vi "Excel Write Full Data Set.vi"(8 "Error In":errorcluster, 9 "CMD Step":dbl format="%#_13g", 10 "Data In":string[][](array[string]), 11 "Cells Ref In":refnum<k7>) -> (0 "Error Out":errorcluster, 3 "Cells Ref Out":refnum<k7>)   [LabVIEW 2013]
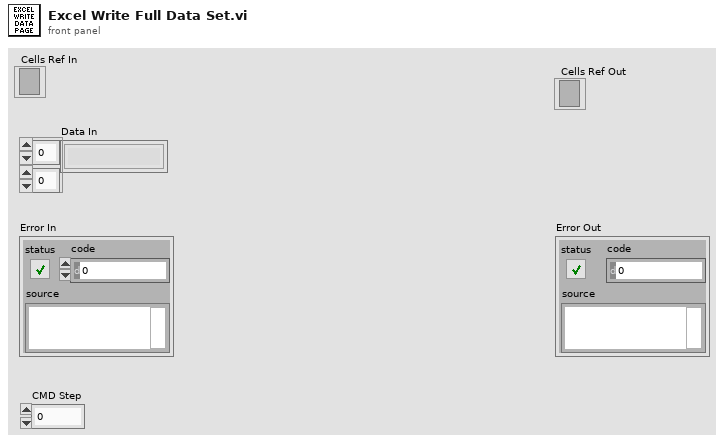
[diagram p1: front panel]
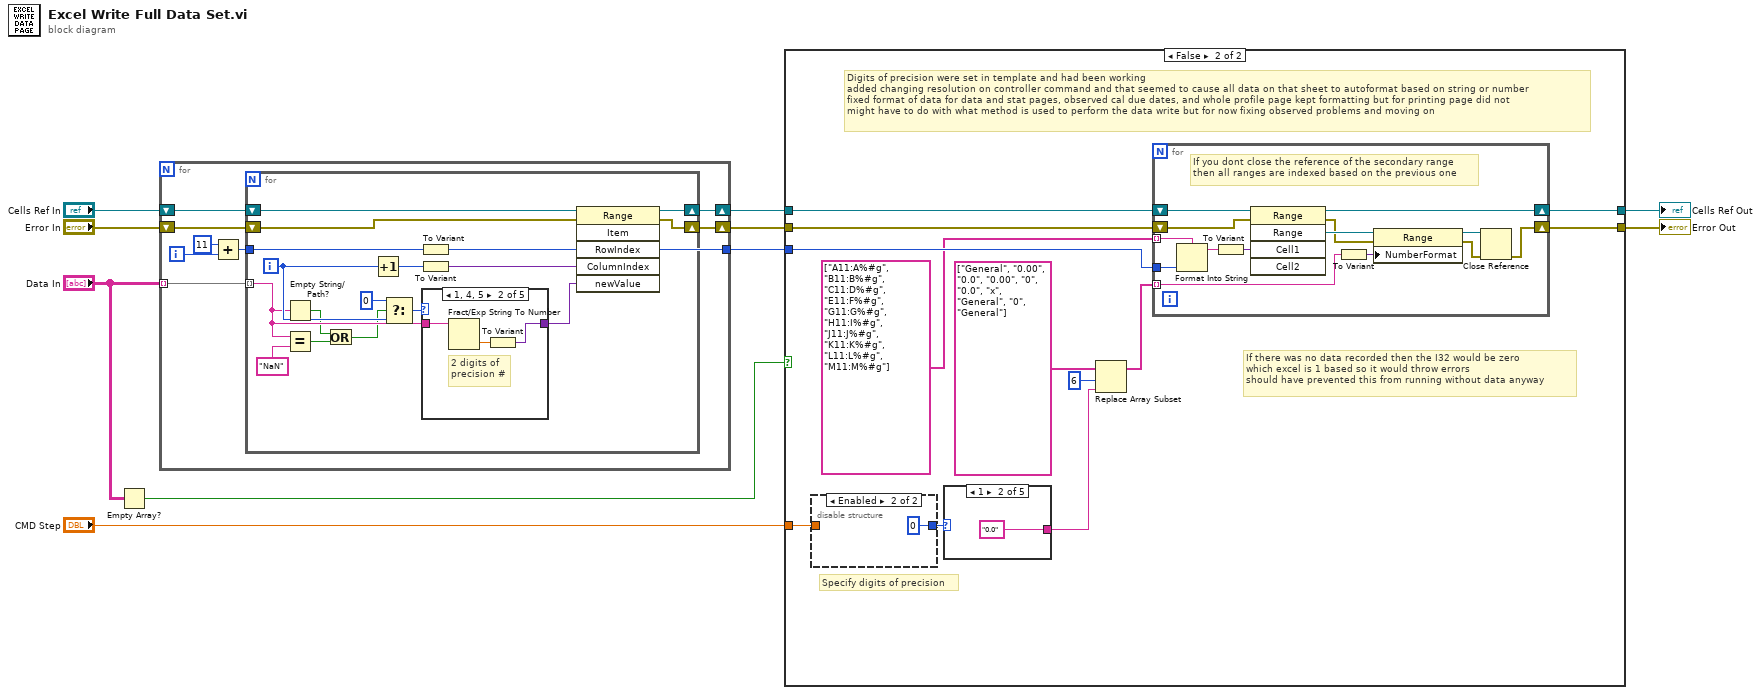
[diagram p0: block diagram]
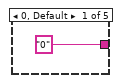
[diagram p4: hidden frame]
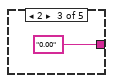
[diagram p5: hidden frame]
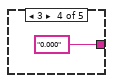
[diagram p6: hidden frame]
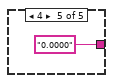
[diagram p7: hidden frame]
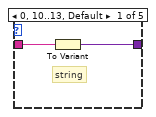
[diagram p8: hidden frame]
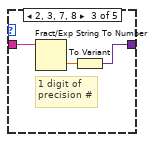
[diagram p9: hidden frame]
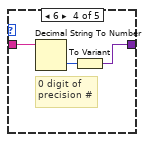
[diagram p10: hidden frame]
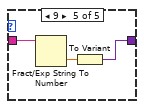
[diagram p11: hidden frame]
diagram:
  n1 = Empty Array?(array="Data In") -> (empty?=w1:bool)
  n2 = for {
    shift-right: [w16] -> w6
    shift-left: "Cells Ref In" -> [w15]
    shift-right: [w17] -> w7
    shift-left: "Error In" -> [w14]
    tunnel: "Data In" -> [w18] mode=indexing
    tunnel: [w11] -> w5
    i -> [w12]
    n3 = Add(x=11, y=w12) -> (x+y=w11:i32)
    n4 = for {
      shift-right: [w20] -> w16
      shift-left: w15 -> [w35]
      shift-right: [w19] -> w17
      shift-left: w14 -> [w34]
      tunnel: w18 -> [w25] mode=indexing
      tunnel: w11 -> [w26]
      i -> [w29]
      n5 = Empty String/Path?(string/path=w25) -> (empty?=w22:bool)
      n6 = Equal?(x=w25, y="NaN") -> (x = y?=w23:bool)
      n7 = Or(x=w22, y=w23) -> (x .or. y?=w21:bool)
      n8 = Increment(x=w29) -> (x+1=w31:i32)
      n9 = Select(t=0, s=w21, f=w29) -> (s? t:f=w27:i32)
      n10 = To Variant(anything=w26) -> (Variant=w33:variant)
      n11 = To Variant(anything=w31) -> (Variant=w32:variant)
      n12 = case shown="1, 4, 5" w27 {
        tunnel: w25 -> [w37 w40 w43 w46 w48]
        tunnel: [w36 w38 w41 w44 w47] -> w30
        frame 0, 10..13, Default {
          # "string"
          n13 = To Variant(anything=w37) -> (Variant=w36:variant)
        }
        frame 1, 4, 5 {
          # "2 digits of\nprecision #"
          n14 = Fract/Exp String To Number(string=w40) -> (number=w39:dbl)  [unwired: 3 in, 1 out]
          n15 = To Variant(anything=w39) -> (Variant=w38:variant)
        }
        frame 2, 3, 7, 8 {
          # "1 digit of\nprecision #"
          n16 = Fract/Exp String To Number(string=w43) -> (number=w42:dbl)  [unwired: 3 in, 1 out]
          n17 = To Variant(anything=w42) -> (Variant=w41:variant)
        }
        frame 6 {
          # "0 digit of\nprecision #"
          n18 = Decimal String To Number(string=w46) -> (number=w45:i32)  [unwired: 2 in, 1 out]
          n19 = To Variant(anything=w45) -> (Variant=w44:variant)
        }
        frame 9 {
          n20 = Fract/Exp String To Number(string=w48) -> (number=w49:dbl)  [unwired: 3 in, 1 out]
          n21 = To Variant(anything=w49) -> (Variant=w47:variant)
        }
      }
      n22 = invoke class="Range" method="Item"(reference=w35, error in=w34, "RowIndex"=w33, "ColumnIndex"=w32, "newValue"=w30) -> (reference out=w20:refnum<k7>, error out=w19:errorcluster)  [unwired: 1 in, 4 out]
    }
  }
  n23 = case shown="False" w1 {
    tunnel: "CMD Step" -> [_ w52]
    tunnel: w7 -> [w50 w63]
    tunnel: w6 -> [w51 w62]
    tunnel: w5 -> [_ w58]
    tunnel: [w51 w57] -> w4
    tunnel: [w50 w56] -> w3
    frame True {
    }
    frame False {
      # "Specify digits of precision"
      # "If there was no data recorded then the I32 would be zero\nwhich excel is 1 based so it would throw errors\nshould have prevented this from running without data anyway"
      # "Digits of precision were set in template and had been working\nadded changing resolution on controller command and that seemed to cause all data on that sheet to autoformat based on string or number\nfixed format of data for data and stat pages, observed cal due dates, and whole profile page kept formatting but for printing page did not\nmight have to do with what method is used to perform the data write but for now fixing observed problems and moving on"
      n24 = disable-structure shown="Enabled" {
        disable-tunnel: [_ 0 ("Digits of Significance")] -> w53
        disable-tunnel: w52 -> [_ _]
        frame Disabled {
        }
        frame Enabled {
        }
      }
      n25 = case shown="1" w53 {
        tunnel: ["0" "0.0" "0.00" "0.000" "0.0000"] -> w59
        frame 0, Default {
        }
        frame 1 {
        }
        frame 2 {
        }
        frame 3 {
        }
        frame 4 {
        }
      }
      n26 = Replace Array Subset(array=string[] ["General", "0.00", "0.0", "0.00", "0", "0.0", "x", "General", "0", "General"], new element=w59, index=6) -> (w55:string[])
      n27 = for {
        shift-right: [w66] -> w57
        shift-left: w62 -> [w72]
        shift-right: [w65] -> w56
        shift-left: w63 -> [w71]
        tunnel: w55 -> [w76] mode=indexing
        tunnel: string[] ["A11:A%#g", "B11:B%#g", "C11:D%#g", "E11:F%#g", "G11:G%#g", "H11:I%#g", "J11:J%#g", "K11:K%#g", "L11:L%#g", "M11:M%#g"] -> [w75] mode=indexing
        tunnel: w58 -> [w74]
        # "If you dont close the reference of the secondary range\nthen all ranges are indexed based on the previous one"
        n28 = Format Into String(format string=w75, w74) -> (resulting string=w78:string)  [unwired: 2 in, 1 out]
        n29 = To Variant(anything=w78) -> (Variant=w73:variant)
        n30 = invoke class="Range" method="Range"(reference=w72, error in=w71, "Cell1"=w73) -> (reference out=w66:refnum<k7>, error out=w69:errorcluster, "Range"=w70:refnum<k7>)  [unwired: 2 in, 2 out]
        n31 = To Variant(anything=w76) -> (Variant=w77:variant)
        n32 = property class="Range"(reference=w70, error in=w69, "NumberFormat"=w77) -> (reference out=w68:refnum<k7>, error out=w67:errorcluster)
        n33 = Close Reference(reference=w68, error in (no error)=w67) -> (error out=w65:errorcluster)
      }
    }
  }
  "Error Out" <- w3
  "Cells Ref Out" <- w4
